vi "MenuOptions.vi"(8 "error in":errorcluster, 9 "VI ref":refnum<vi>, 11 "menu ref in":refnum<k9>) -> (0 "error out":errorcluster, 3 "menu ref out":refnum<k9>)   [LabVIEW 2019, in "Configuration Tool.lvlib"]
doc: "This VI configures the application menu options. If you need aditional menu items add them in this VI."
uses:
  Configuration Tool.lvlib
  <vilib>/Utility/miscctls.llb/LVMenuShortCut.ctl
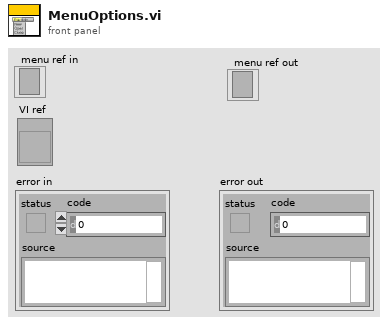
[diagram p1: front panel]
types:
  T1 = typedef "LVMenuShortCut.ctl" = cluster{"Include Shift Key?":bool, "Include Ctrl Key?":bool, "Shortcut Key":string}
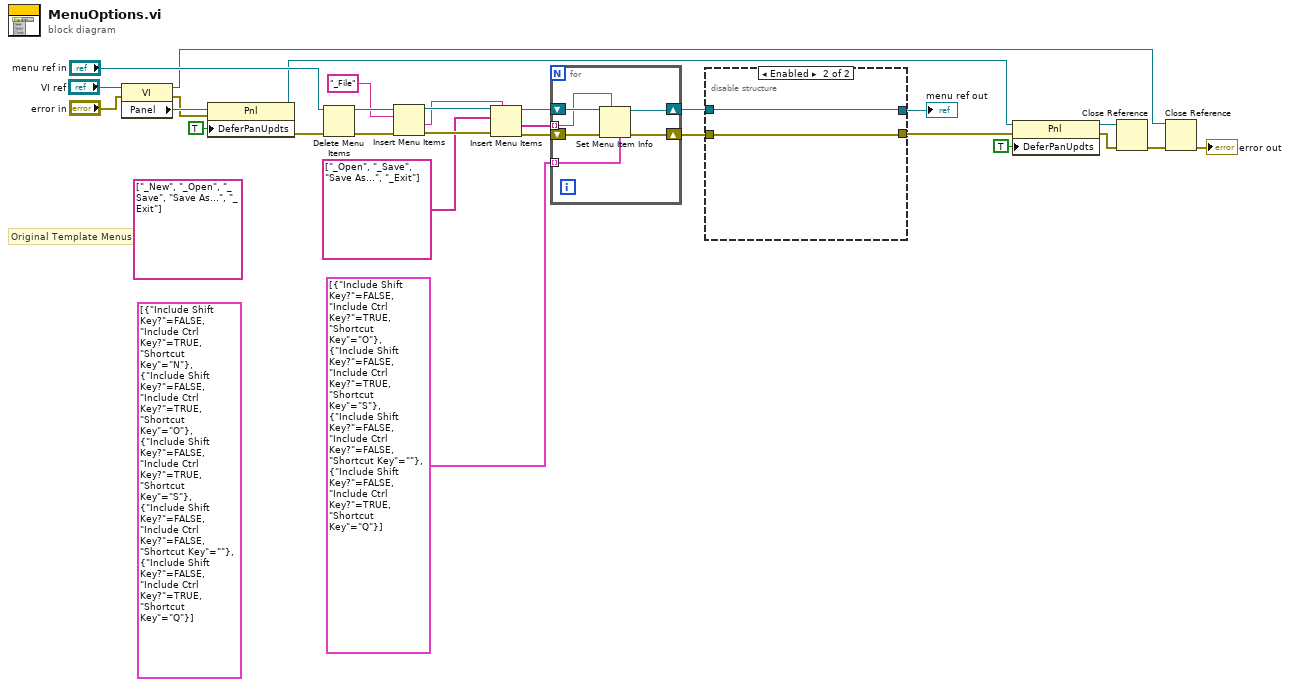
[diagram p0: block diagram]
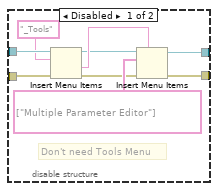
[diagram p2: hidden frame]
diagram:
  (unwired) T1[] [{"Include Shift Key?"=FALSE, "Include Ctrl Key?"=TRUE, "Shortcut Key"="N"}, {"Include Shift Key?"=FALSE, "Include Ctrl Key?"=TRUE, "Shortcut Key"="O"}, {"Include Shift Key?"=FALSE, "Include Ctrl Key?"=TRUE, "Shortcut Key"="S"}, {"Include Shift Key?"=FALSE, "Include Ctrl Key?"=FALSE, "Shortcut Key"=""}, {"Include Shift Key?"=FALSE, "Include Ctrl Key?"=TRUE, "Shortcut Key"="Q"}]
  (unwired) string[] ["_New", "_Open", "_Save", "Save As...", "_Exit"] ("item names")
  # "Original Template Menus"
  n1 = property class="VI"(reference="VI ref", error in="error in") -> (reference out=w15:refnum<vi>, error out=w11:errorcluster, "Panel"=w14:refnum<vi>)
  n2 = property class="Pnl"(reference=w14, error in=w11, "DeferPanUpdts"=TRUE ("Defer Panel Updates")) -> (reference out=w7:refnum<vi>, error out=w10:errorcluster)
  n3 = Delete Menu Items(6:w10, 9:"menu ref in") -> (0:w24:errorcluster, 3:w28:refnum<k9>)  [unwired: 2 in]
  n4 = Insert Menu Items(6:w24, 8:"_File", 9:w28) -> (0:w23:errorcluster, 1:w25:string, 3:w26:refnum<k9>)  [unwired: 3 in]
  n5 = Insert Menu Items(5:w25, 6:w23, 8:string[] ["_Open", "_Save", "Save As...", "_Exit"] ("item names"), 9:w26) -> (0:w21:errorcluster, 1:w20:string[], 3:w22:refnum<k9>)  [unwired: 2 in]
  n6 = for {
    shift-right: [w33] -> w18
    shift-left: w22 -> [w35]
    tunnel: w20 -> [w32] mode=indexing
    tunnel: T1[] [{"Include Shift Key?"=FALSE, "Include Ctrl Key?"=TRUE, "Shortcut Key"="O"}, {"Include Shift Key?"=FALSE, "Include Ctrl Key?"=TRUE, "Shortcut Key"="S"}, {"Include Shift Key?"=FALSE, "Include Ctrl Key?"=FALSE, "Shortcut Key"=""}, {"Include Shift Key?"=FALSE, "Include Ctrl Key?"=TRUE, "Shortcut Key"="Q"}] -> [w30] mode=indexing
    shift-right: [w31] -> w17
    shift-left: w21 -> [w34]
    n7 = Set Menu Item Info(4:w30, 7:w32, 8:w34, 11:w35) -> (0:w31:errorcluster, 3:w33:refnum<k9>)  [unwired: 3 in]
  }
  n8 = disable-structure shown="Enabled" {
    disable-tunnel: [w44 w46] -> w19
    disable-tunnel: w18 -> [w43 w46]
    disable-tunnel: w17 -> [w42 w45]
    disable-tunnel: [w36 w45] -> w8
    frame Disabled {
      # "Don't need Tools Menu"
      n9 = Insert Menu Items(6:w42, 8:"_Tools", 9:w43) -> (0:w39:errorcluster, 1:w41:string, 3:w38:refnum<k9>)  [unwired: 3 in]
      n10 = Insert Menu Items(5:w41, 6:w39, 8:string[] ["Multiple Parameter Editor"] ("item names"), 9:w38) -> (0:w36:errorcluster, 3:w44:refnum<k9>)  [unwired: 2 in, 1 out]
    }
    frame Enabled {
    }
  }
  "menu ref out" <- w19
  n11 = property class="Pnl"(reference=w7, error in=w8, "DeferPanUpdts"=TRUE ("Defer Panel Updates")) -> (reference out=w6:refnum<vi>, error out=w5:errorcluster)
  n12 = Close Reference(reference=w6, error in (no error)=w5) -> (error out=w4:errorcluster)
  n13 = Close Reference(reference=w15, error in (no error)=w4) -> (error out=→"error out":errorcluster)
